vi "BaseProvider_PlugInManager.vi"(1 "PlugInName":string, 2 "ClassRefToActOn":refnum<vi>, 3 "ExtraExInfo":string, 4 "PlugInPath":path, 5 "error in (no error)":errorcluster, 6 "Action":T1) -> (15 "MethodsTypes":string[](array[string]), 19 "error out":errorcluster)   [LabVIEW 2020]
uses:
  <resource>/Framework/Providers/Open_GDS/ClassProviders/Provider_BaseClassInterface/BaseProvider_SubVIs/BaseProvider_PlugInManagerActions.ctl
panel:
  in  "PlugInInterface":refnum<vi>
  out "DummyError":errorcluster
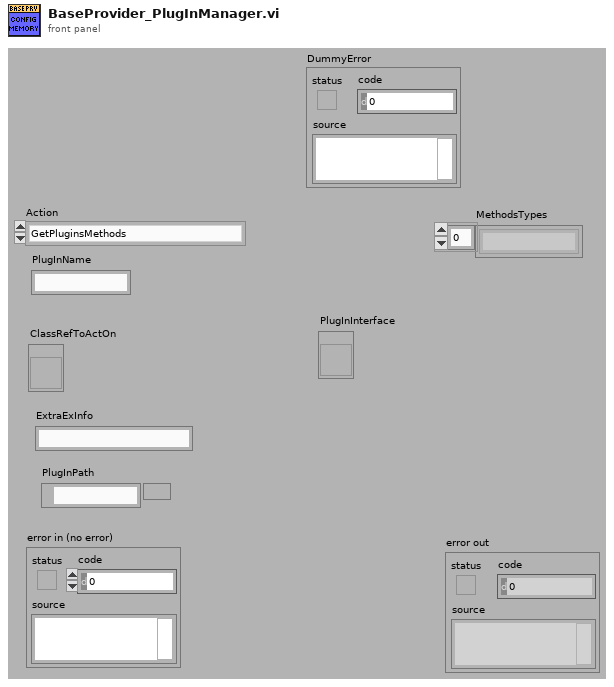
[diagram p1: front panel]
types:
  T1 = typedef "BaseProvider_PlugInManagerActions.ctl" = enum16{"GetPluginsMethods", "ExecutePlugIn"}
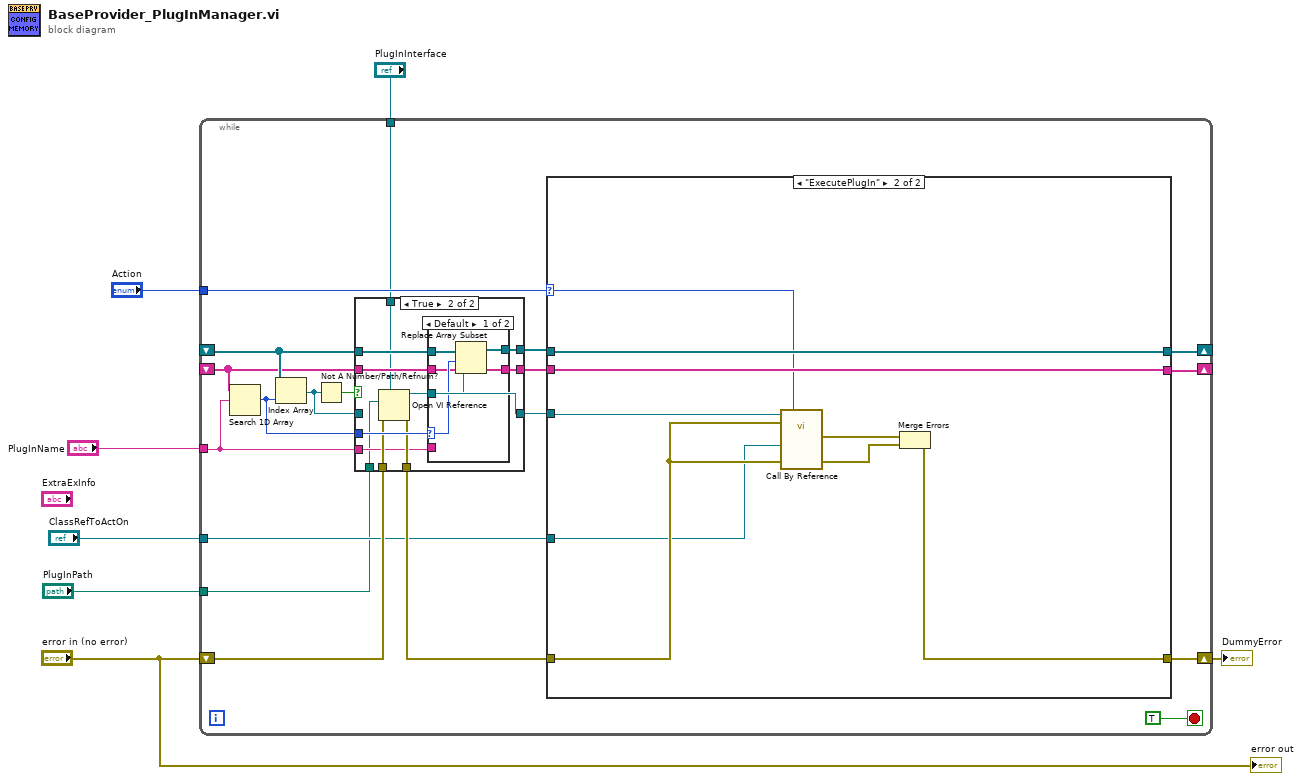
[diagram p0: block diagram]
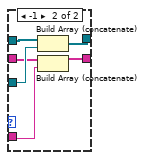
[diagram p3: hidden frame]
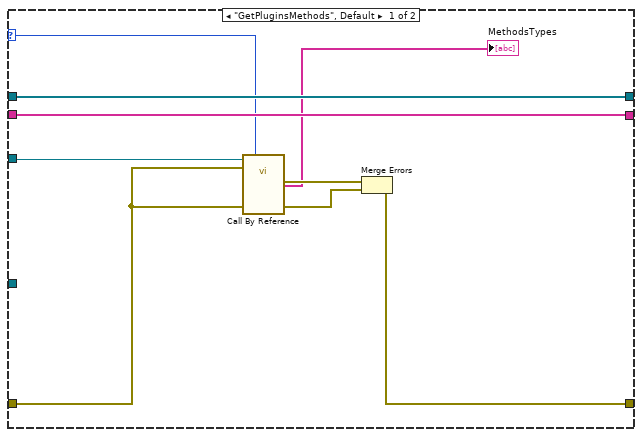
[diagram p4: hidden frame]
diagram:
  n1 = while {
    tunnel: "Action" -> [w26]
    shift-right: [w24] -> _
    shift-left: _ -> [w20]
    shift-right: [w23] -> _
    shift-left: _ -> [w18]
    tunnel: "PlugInName" -> [w10]
    shift-right: [w11] -> w5
    shift-left: "error in (no error)" -> [w16]
    tunnel: "PlugInInterface" -> [w12]
    tunnel: "ClassRefToActOn" -> [w9]
    tunnel: "PlugInPath" -> [w8]
    stop <- TRUE stop-if-true
    n2 = Search 1D Array(1D array=w18, element=w10) -> (index of element=w21:i32)  [unwired: 1 in]
    n3 = Index Array(array=w20, index=w21) -> (element=w15:refnum<vi>)
    n4 = Not A Number/Path/Refnum?(number/path/refnum=w15) -> (NaN/Path/Refnum?=w22:bool)
    n5 = case shown="True" w22 {
      tunnel: w21 -> [_ w41]
      tunnel: w20 -> [w29 w40]
      tunnel: [w29 w39] -> w19
      tunnel: w18 -> [w28 w38]
      tunnel: [w28 w37] -> w17
      tunnel: w16 -> [w30 w36]
      tunnel: [w30 w35] -> w13
      tunnel: w10 -> [_ w34]
      tunnel: w15 -> [w27 _]
      tunnel: [w27 w33] -> w14
      tunnel: w12 -> [_ w32]
      tunnel: w8 -> [_ w31]
      frame False {
      }
      frame True {
        n6 = Open VI Reference(type specifier VI Refnum (for type only)=w32, vi path=w31, error in (no error)=w36) -> (vi reference=w33:refnum<vi>, error out=w35:errorcluster)  [unwired: 3 in]
        n7 = case shown="Default" w41 {
          selector: w41 -> [w44 _]
          tunnel: w40 -> [w45 w47]
          tunnel: [w46 w52] -> w39
          tunnel: w38 -> [w43 w48]
          tunnel: [w43 w51] -> w37
          tunnel: w33 -> [w42 w50]
          tunnel: w34 -> [_ w49]
          frame Default {
            n8 = Replace Array Subset(array=w45, new element=w42, index=w44) -> (w46:refnum<vi>[])
          }
          frame -1 {
            n9 = Build Array (concatenate)(w47, w50) -> (w52:refnum<vi>[])
            n10 = Build Array (concatenate)(w48, w49) -> (w51:string[])
          }
        }
      }
    }
    n11 = case shown="\"ExecutePlugIn\"" w26 {
      selector: w26 -> [w53 w63]
      tunnel: [w61 w70] -> w24
      tunnel: [w60 w69] -> w23
      tunnel: w19 -> [w61 w70]
      tunnel: w17 -> [w60 w69]
      tunnel: w14 -> [w59 w68]
      tunnel: w13 -> [w58 w67]
      tunnel: [w55 w64] -> w11
      tunnel: w9 -> [_ w62]
      frame "GetPluginsMethods", Default {
        n12 = call-by-ref "?"(reference=w59, error in=w58, 5:"error in (no error)"=w58, "Action"=w53) -> (error out=w56:errorcluster, "MethodsTypes"=→"MethodsTypes":string[], 19:"error out"=w57:errorcluster)  [unwired: 16 in, 1 out]
        n13 = Merge Errors(w56, w57) -> (w55:errorcluster)
      }
      frame "ExecutePlugIn" {
        n14 = call-by-ref "?"(reference=w68, error in=w67, "ClassRefToActOn"=w62, 5:"error in (no error)"=w67, "Action"=w63) -> (error out=w65:errorcluster, 19:"error out"=w66:errorcluster)  [unwired: 15 in, 2 out]
        n15 = Merge Errors(w65, w66) -> (w64:errorcluster)
      }
    }
  }
  "DummyError" <- w5
  "error out" <- "error in (no error)"
